vi "R1Initialize.vi"(8 "error in (no error)":errorcluster) -> (0 "error out":errorcluster)   [LabVIEW 2016]
uses:
  Controls/R1SBR_SetParams.ctl
  Controls/pH_SetParams Standard.ctl
  Controls/ISE_CF.ctl
  Controls/pH_Manual Standard.ctl
panel:
  out "?":dbl
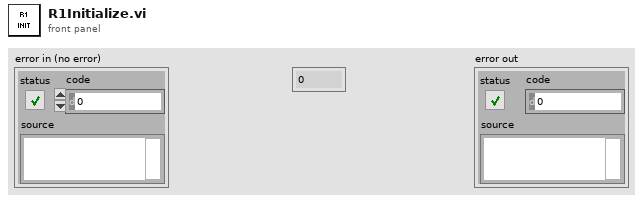
[diagram p1: front panel]
types:
  T1 = typedef "ISE_CF.ctl" = cluster{"Correction Factor":dbl, "Ion":string, "Correct For Ion?":bool}
  T2 = cluster{"Equil Approach Set point, mV/min":dbl, "Equil Approach dt, s":dbl, "Interference Correction Factors":T1[], "Detect Equilibrium?":bool, "Probe Intercept":dbl, "Probe Slope":dbl, "Baseline":dbl, "Detection Limit, M":dbl}
  T3 = cluster{"Media Pump":bool, "Water Pump":bool, "Effluent Pump":bool, "Release Valve":bool, "Gas Pump":bool}
  T4 = cluster{"Set Point, mg/L":dbl, "Tolerance, mg/L":dbl, "N2 Valve Gain":dbl, "Air Valve Gain":dbl}
  T5 = typedef "pH_SetParams Standard.ctl" = cluster{"Set Point":dbl, "Tolerance":dbl, "Pump Time On, secs":dbl}
  T6 = typedef "R1SBR_SetParams.ctl" = cluster{"Phase":string, "Time, min":dbl, "SBR_Manual":cluster{"Media Pump":bool, "Water Pump":bool, "Effluent Pump":bool, "Release Valve":bool, "Gas Pump":bool}}[]
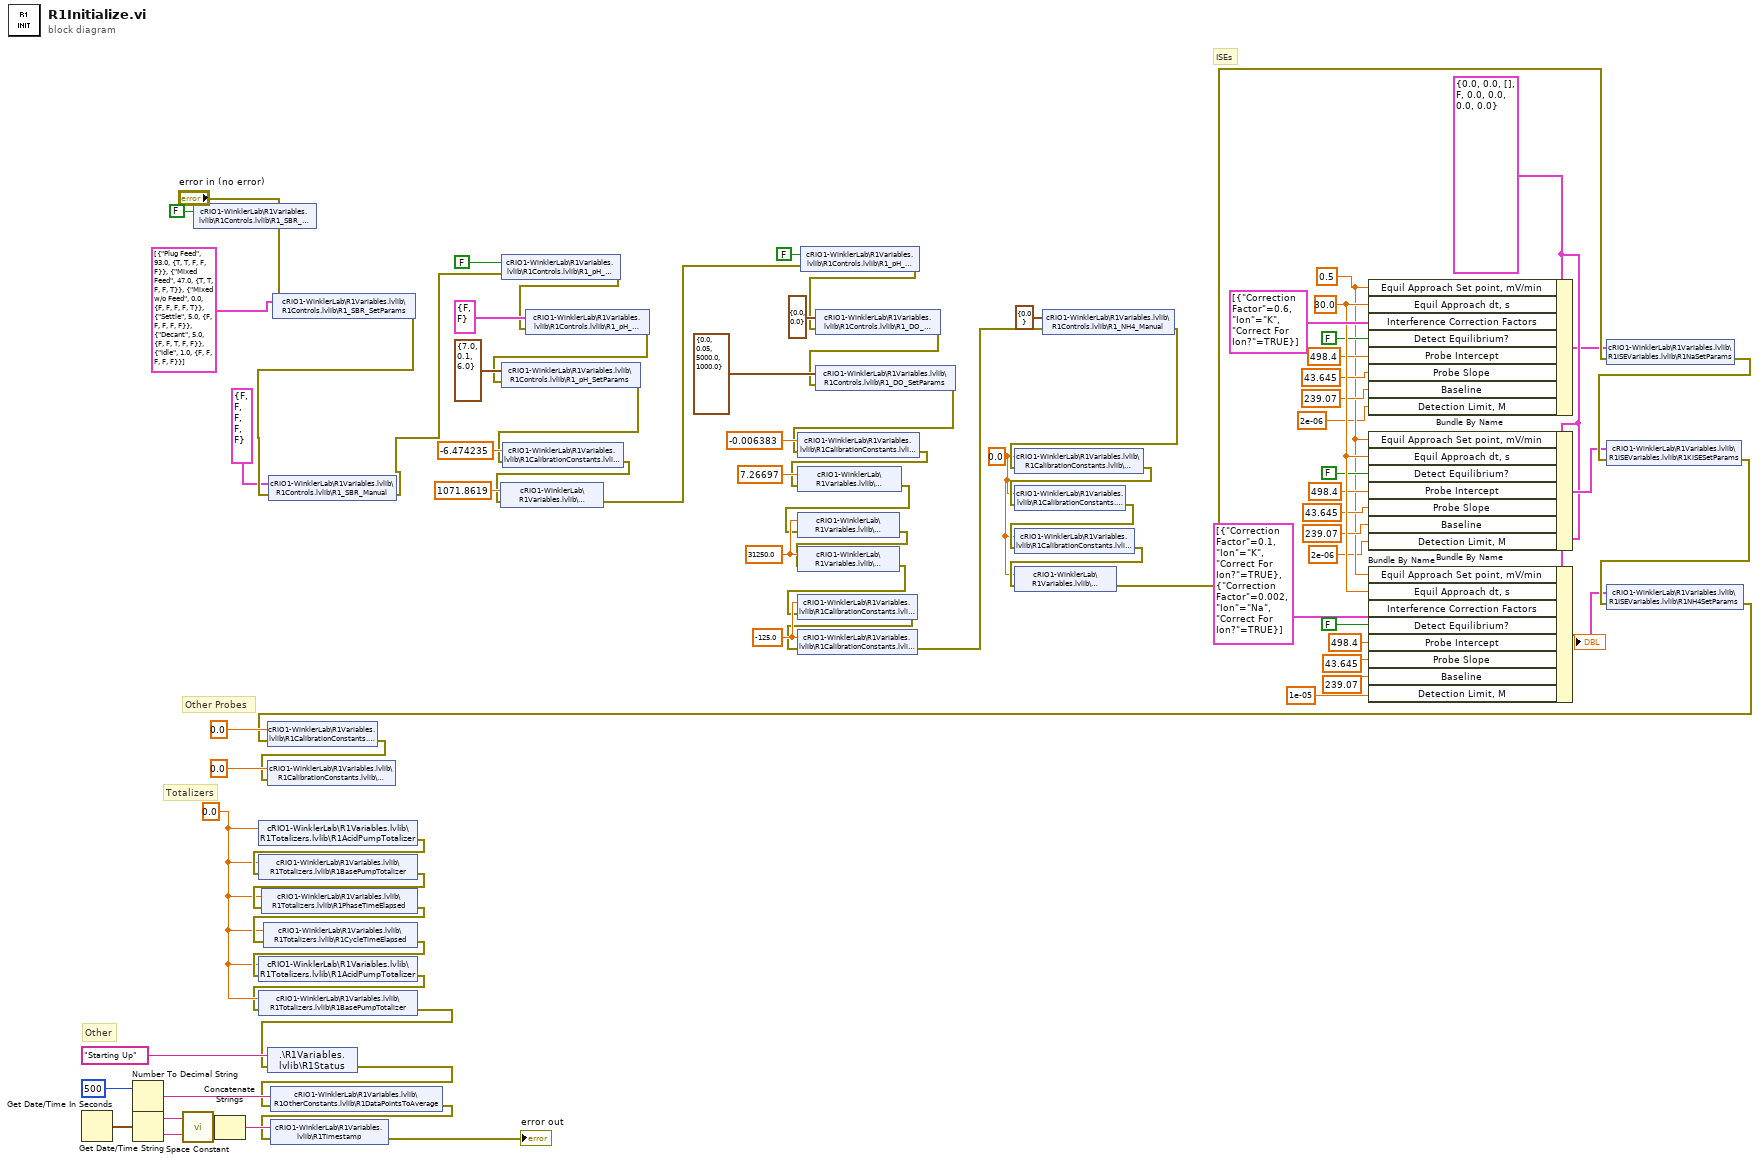
[diagram p0: block diagram]
diagram:
  w5 = T2 {"Equil Approach Set point, mV/min"=0.0, "Equil Approach dt, s"=0.0, "Interference Correction Factors"=[], "Detect Equilibrium?"=FALSE, "Probe Intercept"=0.0, "Probe Slope"=0.0, "Baseline"=0.0, "Detection Limit, M"=0.0} ("R1NaSetParams")
  w26 = 30.0 ("Equil Approach dt, s")
  w6 = 0.5 ("Equil Approach Set point, mV/min")
  w31 = 0.0 ("R1NH4Intercept")
  w41 = 0.0 ("R1PhaseTimeElapsed")
  w71 = 31250.0 ("R1AirSlope")
  w72 = -125.0 ("R1N2Intercept")
  # "ISEs"
  # "Totalizers"
  # "Other Probes"
  # "Other"
  n1 = Get Date/Time In Seconds() -> (seconds since 1Jan1904=w50:timestamp)
  n2 = Number To Decimal String(number=500 ("R1DataPointsToAverage")) -> (decimal integer string=w77:string)  [unwired: 1 in]
  n3 = Get Date/Time String(seconds (now)=w50) -> (date string=w38:string, time string=w49:string)  [unwired: 2 in]
  n4 = call <vilib>:"Space Constant.vi"() -> ("String"=w48:string)
  n5 = shared-variable "cRIO1-WinklerLab\\R1Variables.lvlib\\R1Controls.lvlib\\R1_SBR_Switch"(FALSE ("R1SBRSwitch")) -> ()  [unwired: 1 in, 1 out]
  n6 = Concatenate Strings(w38, w48, w49) -> (w46:string)
  n7 = shared-variable "cRIO1-WinklerLab\\R1Variables.lvlib\\R1Totalizers.lvlib\\R1AcidPumpTotalizer"(w41) -> (error out=w43:errorcluster)  [unwired: 1 in]
  n8 = shared-variable "cRIO1-WinklerLab\\R1Variables.lvlib\\R1Totalizers.lvlib\\R1BasePumpTotalizer"(w41, error in=w43) -> (error out=w44:errorcluster)
  n9 = shared-variable "cRIO1-WinklerLab\\R1Variables.lvlib\\R1Totalizers.lvlib\\R1PhaseTimeElapsed"(w41, error in=w44) -> (error out=w51:errorcluster)
  n10 = shared-variable "cRIO1-WinklerLab\\R1Variables.lvlib\\R1Totalizers.lvlib\\R1CycleTimeElapsed"(w41, error in=w51) -> (error out=w42:errorcluster)
  n11 = shared-variable "cRIO1-WinklerLab\\R1Variables.lvlib\\R1Totalizers.lvlib\\R1AcidPumpTotalizer"(w41, error in=w42) -> (error out=w40:errorcluster)
  n12 = shared-variable "cRIO1-WinklerLab\\R1Variables.lvlib\\R1Totalizers.lvlib\\R1BasePumpTotalizer"(w41, error in=w40) -> (error out=w39:errorcluster)
  n13 = shared-variable ".\\R1Variables.lvlib\\R1Status"("Starting Up" ("R1Status"), error in=w39) -> (error out=w53:errorcluster)
  n14 = shared-variable "cRIO1-WinklerLab\\R1Variables.lvlib\\R1OtherConstants.lvlib\\R1DataPointsToAverage"(w77, error in=w53) -> (error out=w45:errorcluster)
  n15 = shared-variable "cRIO1-WinklerLab\\R1Variables.lvlib\\R1Timestamp"(w46, error in=w45) -> (error out=→"error out":errorcluster)
  n16 = shared-variable "cRIO1-WinklerLab\\R1Variables.lvlib\\R1Controls.lvlib\\R1_SBR_SetParams"(T6 [{"Phase"="Plug Feed", "Time, min"=93.0, "SBR_Manual"={"Media Pump"=TRUE, "Water Pump"=TRUE, "Effluent Pump"=FALSE, "Release Valve"=FALSE, "Gas Pump"=FALSE}}, {"Phase"="Mixed Feed", "Time, min"=47.0, "SBR_Manual"={"Media Pump"=TRUE, "Water Pump"=TRUE, "Effluent Pump"=FALSE, "Release Valve"=FALSE, "Gas Pump"=TRUE}}, {"Phase"="Mixed w/o Feed", "Time, min"=0.0, "SBR_Manual"={"Media Pump"=FALSE, "Water Pump"=FALSE, "Effluent Pump"=FALSE, "Release Valve"=FALSE, "Gas Pump"=TRUE}}, {"Phase"="Settle", "Time, min"=5.0, "SBR_Manual"={"Media Pump"=FALSE, "Water Pump"=FALSE, "Effluent Pump"=FALSE, "Release Valve"=FALSE, "Gas Pump"=FALSE}}, {"Phase"="Decant", "Time, min"=5.0, "SBR_Manual"={"Media Pump"=FALSE, "Water Pump"=FALSE, "Effluent Pump"=TRUE, "Release Valve"=FALSE, "Gas Pump"=FALSE}}, {"Phase"="Idle", "Time, min"=1.0, "SBR_Manual"={"Media Pump"=FALSE, "Water Pump"=FALSE, "Effluent Pump"=FALSE, "Release Valve"=FALSE, "Gas Pump"=FALSE}}] ("R1SBR_SetParams 2"), error in="error in (no error)") -> (error out=w30:errorcluster)
  n17 = shared-variable "cRIO1-WinklerLab\\R1Variables.lvlib\\R1Controls.lvlib\\R1_SBR_Manual"(T3 {"Media Pump"=FALSE, "Water Pump"=FALSE, "Effluent Pump"=FALSE, "Release Valve"=FALSE, "Gas Pump"=FALSE} ("R1SBRManual"), error in=w30) -> (error out=w28:errorcluster)
  n18 = shared-variable "cRIO1-WinklerLab\\R1Variables.lvlib\\R1Controls.lvlib\\R1_pH_Switch"(FALSE ("R1pHSwitch"), error in=w28) -> (error out=w67:errorcluster)
  n19 = shared-variable "cRIO1-WinklerLab\\R1Variables.lvlib\\R1Controls.lvlib\\R1_pH_Manual"(cluster{"Acid Pump":bool, "Base Pump":bool} {"Acid Pump"=FALSE, "Base Pump"=FALSE} ("R1pHManual"), error in=w67) -> (error out=w66:errorcluster)
  n20 = shared-variable "cRIO1-WinklerLab\\R1Variables.lvlib\\R1Controls.lvlib\\R1_pH_SetParams"(T5 {"Set Point"=7.0, "Tolerance"=0.1, "Pump Time On, secs"=6.0} ("R1pHSetParams"), error in=w66) -> (error out=w65:errorcluster)
  n21 = shared-variable "cRIO1-WinklerLab\\R1Variables.lvlib\\R1CalibrationConstants.lvlib\\R1pHIntercept"(-6.474235 ("R12pHInt"), error in=w65) -> (error out=w62:errorcluster)
  n22 = shared-variable "cRIO1-WinklerLab\\R1Variables.lvlib\\R1CalibrationConstants.lvlib\\R1pHSlope"(1071.8619 ("R1pHSlope"), error in=w62) -> (error out=w63:errorcluster)
  n23 = shared-variable "cRIO1-WinklerLab\\R1Variables.lvlib\\R1Controls.lvlib\\R1_pH_Switch"(FALSE ("R1pHSwitch"), error in=w63) -> (error out=w61:errorcluster)
  n24 = shared-variable "cRIO1-WinklerLab\\R1Variables.lvlib\\R1Controls.lvlib\\R1_DO_Manual"(cluster{"Air MFC":dbl, "N2 MFC":dbl} {"Air MFC"=0.0, "N2 MFC"=0.0} ("R1DOManual"), error in=w61) -> (error out=w60:errorcluster)
  n25 = shared-variable "cRIO1-WinklerLab\\R1Variables.lvlib\\R1Controls.lvlib\\R1_DO_SetParams"(T4 {"Set Point, mg/L"=0.0, "Tolerance, mg/L"=0.05, "N2 Valve Gain"=5000.0, "Air Valve Gain"=1000.0} ("R1DOSetParams"), error in=w60) -> (error out=w59:errorcluster)
  n26 = shared-variable "cRIO1-WinklerLab\\R1Variables.lvlib\\R1CalibrationConstants.lvlib\\R1DOIntercept"(-0.006383 ("R1DOInt"), error in=w59) -> (error out=w58:errorcluster)
  n27 = shared-variable "cRIO1-WinklerLab\\R1Variables.lvlib\\R1CalibrationConstants.lvlib\\R1DOSlope"(7.26697 ("R1DOSlope"), error in=w58) -> (error out=w57:errorcluster)
  n28 = shared-variable "cRIO1-WinklerLab\\R1Variables.lvlib\\R1CalibrationConstants.lvlib\\R1N2Slope"(w71, error in=w57) -> (error out=w56:errorcluster)
  n29 = shared-variable "cRIO1-WinklerLab\\R1Variables.lvlib\\R1CalibrationConstants.lvlib\\R1AirSlope"(w71, error in=w56) -> (error out=w55:errorcluster)
  n30 = shared-variable "cRIO1-WinklerLab\\R1Variables.lvlib\\R1CalibrationConstants.lvlib\\R1AirIntercept"(w72, error in=w55) -> (error out=w54:errorcluster)
  n31 = shared-variable "cRIO1-WinklerLab\\R1Variables.lvlib\\R1CalibrationConstants.lvlib\\R1N2Intercept"(w72, error in=w54) -> (error out=w36:errorcluster)
  n32 = shared-variable "cRIO1-WinklerLab\\R1Variables.lvlib\\R1Controls.lvlib\\R1_NH4_Manual"(cluster{"NH4 Pump Flowrate, ml/min":dbl} {"NH4 Pump Flowrate, ml/min"=0.0} ("R1NH4Manual"), error in=w36) -> (error out=w35:errorcluster)
  n33 = shared-variable "cRIO1-WinklerLab\\R1Variables.lvlib\\R1CalibrationConstants.lvlib\\R1NH4Intercept"(w31, error in=w35) -> (error out=w32:errorcluster)
  n34 = shared-variable "cRIO1-WinklerLab\\R1Variables.lvlib\\R1CalibrationConstants.lvlib\\R1NH4Slope"(w31, error in=w32) -> (error out=w34:errorcluster)
  n35 = shared-variable "cRIO1-WinklerLab\\R1Variables.lvlib\\R1CalibrationConstants.lvlib\\R1NaIntercept"(w31, error in=w34) -> (error out=w33:errorcluster)
  n36 = shared-variable "cRIO1-WinklerLab\\R1Variables.lvlib\\R1CalibrationConstants.lvlib\\R1NaSlope"(w31, error in=w33) -> (error out=w24:errorcluster)
  n37 = Bundle By Name(cluster=w5, "Equil Approach Set point, mV/min"=w6, "Equil Approach dt, s"=w26, "Interference Correction Factors"=T1[] [{"Correction Factor"=0.6, "Ion"="K", "Correct For Ion?"=TRUE}], "Detect Equilibrium?"=FALSE, "Probe Intercept"=498.4, "Probe Slope"=43.645 ("Equil Approach dt, s"), "Baseline"=239.07 ("Equil Approach dt, s"), "Detection Limit, M"=2e-06) -> (w2:T2)
  n38 = Bundle By Name(cluster=w5, "Equil Approach Set point, mV/min"=w6, "Equil Approach dt, s"=w26, "Detect Equilibrium?"=FALSE, "Probe Intercept"=498.4, "Probe Slope"=43.645 ("Equil Approach dt, s"), "Baseline"=239.07 ("Equil Approach dt, s"), "Detection Limit, M"=2e-06) -> (w20:T2)
  n39 = Bundle By Name(cluster=w5, "Equil Approach Set point, mV/min"=w6, "Equil Approach dt, s"=w26, "Interference Correction Factors"=T1[] [{"Correction Factor"=0.1, "Ion"="K", "Correct For Ion?"=TRUE}, {"Correction Factor"=0.002, "Ion"="Na", "Correct For Ion?"=TRUE}], "Detect Equilibrium?"=FALSE, "Probe Intercept"=498.4, "Probe Slope"=43.645 ("Equil Approach dt, s"), "Baseline"=239.07 ("Equil Approach dt, s"), "Detection Limit, M"=1e-05) -> (w19:T2)
  n40 = shared-variable "cRIO1-WinklerLab\\R1Variables.lvlib\\R1ISEVariables.lvlib\\R1NaSetParams"(w2, error in=w24) -> (error out=w23:errorcluster)
  n41 = shared-variable "cRIO1-WinklerLab\\R1Variables.lvlib\\R1ISEVariables.lvlib\\R1KISESetParams"(w20, error in=w23) -> (error out=w22:errorcluster)
  n42 = shared-variable "cRIO1-WinklerLab\\R1Variables.lvlib\\R1ISEVariables.lvlib\\R1NH4SetParams"(w19, error in=w22) -> (error out=w21:errorcluster)
  n43 = shared-variable "cRIO1-WinklerLab\\R1Variables.lvlib\\R1CalibrationConstants.lvlib\\R1ORPSlope"(0.0 ("R1ORPSlope"), error in=w21) -> (error out=w52:errorcluster)
  n44 = shared-variable "cRIO1-WinklerLab\\R1Variables.lvlib\\R1CalibrationConstants.lvlib\\R1ORPIntercept"(0.0 ("R1ORPIntercept"), error in=w52) -> ()  [unwired: 1 out]
